vi "Monitoring task.vi"   [LabVIEW 2016]
uses:
  PLC/PLC.lvlib
types:
  T1 = enum16{"启动测量", "标样核查", "零点核查", "跨度核查", "空白测试", "平行样测试", "加标回收", "空白校准", "标样校准", "初始化（清洗）", "停止测试", "仪器重启", "校时", "模式设置", "测量间隔设置"}
  T2 = cluster{"参数启用":cluster{"氨氮":bool, "总磷":bool, "总氮":bool, "多参数":bool, "CODMn":bool, "CODcr":bool, "超标留样":bool}}
  T3 = cluster{"时间标识":timestamp, "设备":string, "日志信息":string, "流程参数":string}
  T4 = cluster{"测量模式":enum16{"水样测量", "标样核查", "零点核查", "跨度核查", "空白测试", "加标回收", "平行样", "校零", "校标"}}
  T5 = cluster{"时间标识":timestamp, "设备":string, "日志信息":string}
  T6 = enum16{"空闲", "水样测试", "标样核查", "零点核查", "跨度核查", "空白测试", "平行样测试", "加标回收", "空白校准", "标样校准", "初始化（清洗）"}
  T7 = cluster{"系统时间":timestamp, "工作状态":u16, "测量模式":enum16{"待机", "连续模式", "周期模式", "定点模式", "受控模式", "手动模式"}, "告警代码":u16, "故障代码":u16, "日志代码":u16, "软件版本":u16, "F0":sgl, "F1":sgl, "F2":sgl, "F3":sgl, "T":sgl, "H":sgl, "id":u16, "flowid":u16, "量程":u16, "总磷控温温度1":sgl, "营养盐控温温度2":sgl, "ADC":sgl}
  T8 = enum16{"空闲", "水样测试", "标样核查", "零点核查", "跨度核查", "空白测试", "平行样测试", "质控样", "空白校准", "标样校准", "加标回收"}
  T9 = enum32{"Bad", "Idle", "Run top level", "Running"}
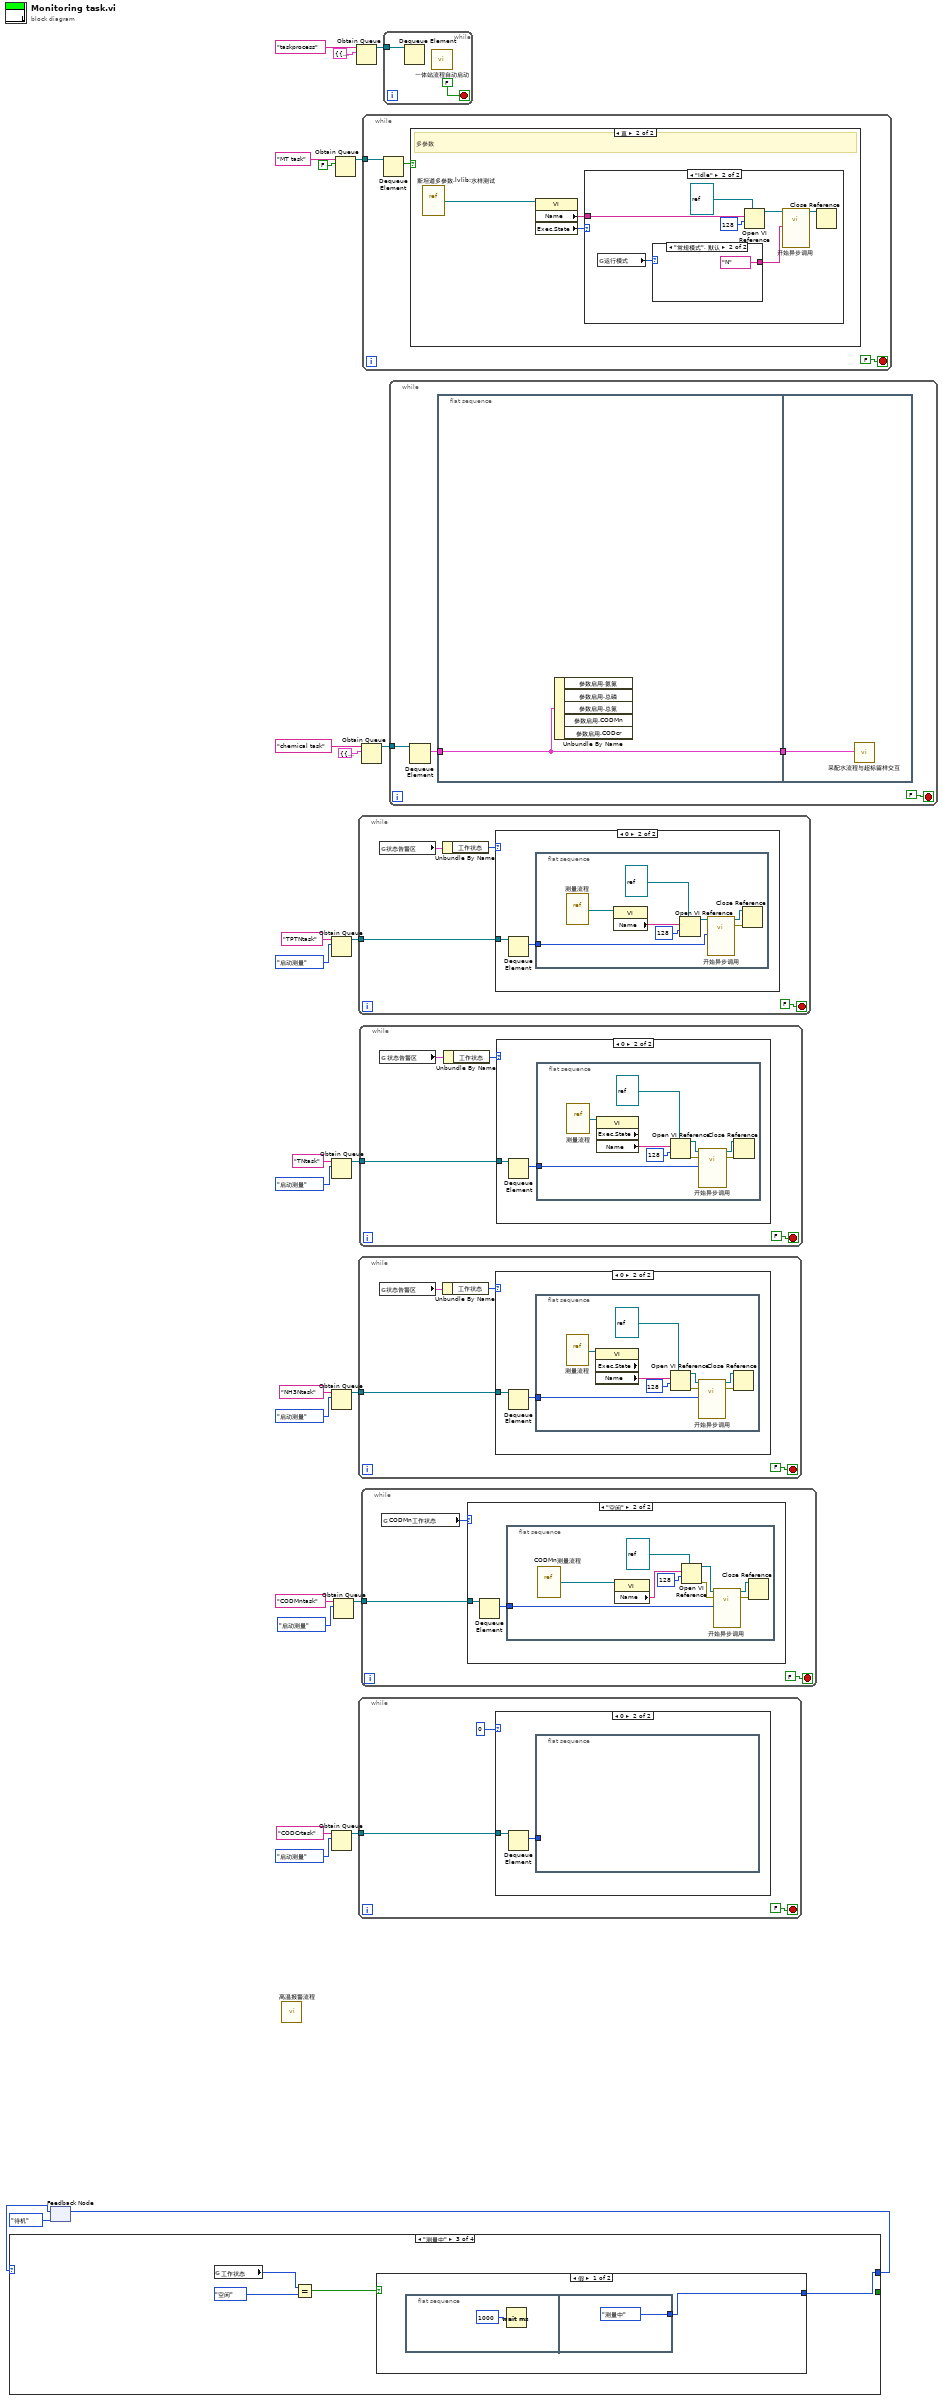
[diagram p0: block diagram]
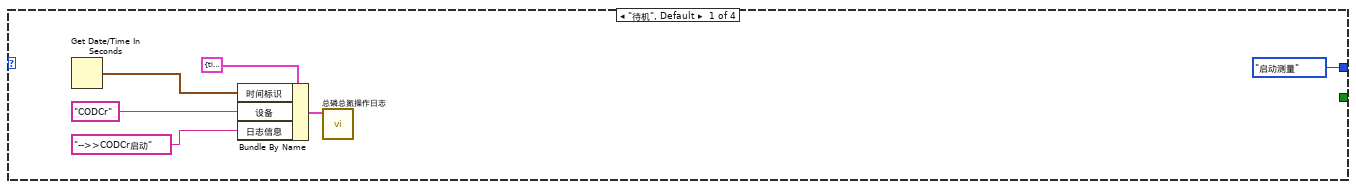
[diagram p2: hidden frame]
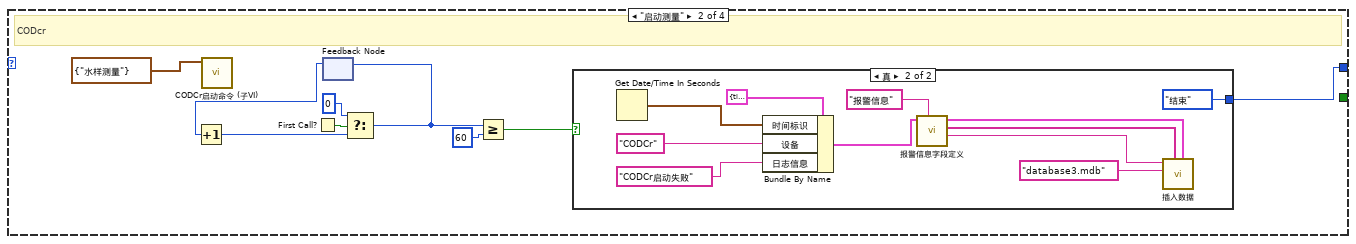
[diagram p3: hidden frame]
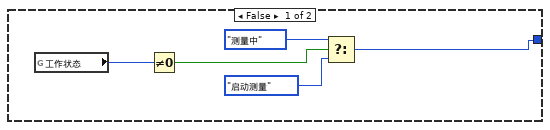
[diagram p4: hidden frame]
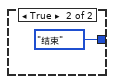
[diagram p5: hidden frame]
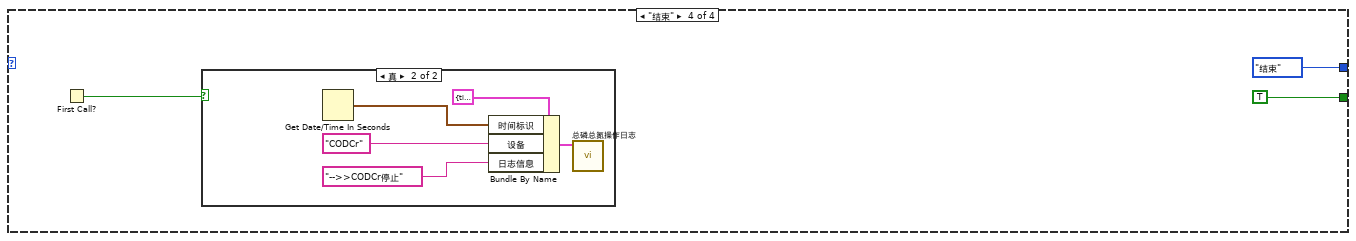
[diagram p6: hidden frame]
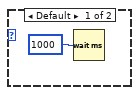
[diagram p8: hidden frame]
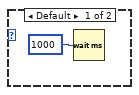
[diagram p9: hidden frame]
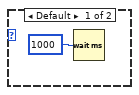
[diagram p10: hidden frame]
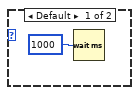
[diagram p11: hidden frame]
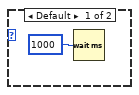
[diagram p12: hidden frame]
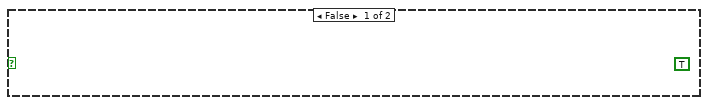
[diagram p13: hidden frame]
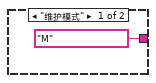
[diagram p15: hidden frame]
diagram:
  n1 = feedback #1(enum16{"待机", "启动测量", "测量中", "结束"}."待机") -> (w2:enum16{"待机", "启动测量", "测量中", "结束"})
  n2 = case shown="\"测量中\"" w2 {
    tunnel: [enum16{"待机", "启动测量", "测量中", "结束"}."启动测量" w42 w62 enum16{"待机", "启动测量", "测量中", "结束"}."结束"] -> w1
    tunnel: [_ _ _ TRUE] -> _
    frame "待机", Default {
      n3 = Get Date/Time In Seconds() -> (seconds since 1Jan1904=w32:timestamp)
      n4 = Bundle By Name(cluster=T3 {"时间标识"=timestamp(0 s since 1904-01-01), "设备"="", "日志信息"="", "流程参数"=""} ("data in"), "时间标识"=w32, "设备"="CODCr", "日志信息"="-->>CODCr启动") -> (w28:T3)
      n5 = call "总磷总氮操作日志.vi"("data in"=w28) -> ()  [unwired: 11 in]
    }
    frame "启动测量" {
      # "CODcr"
      n6 = call "CODCr启动命令 (子VI).vi"("启动测量模式"=T4 {"测量模式"=enum."水样测量"}) -> ()  [unwired: 11 in]
      n7 = First Call?() -> (First Call?: T/F=w37:bool)
      n8 = feedback #2() -> (w38:i32)  [unwired: 1 in]
      n9 = Increment(x=w38) -> (x+1=w39:i32)
      n10 = Select(t=0, s=w37, f=w39) -> (s? t:f=w40:i32)
      n11 = feedback-in #2(w40) -> ()
      n12 = Greater Or Equal?(x=w40, y=60) -> (x >= y?=w35:bool)
      n13 = case shown="真" w35 {
        tunnel: [w43 enum16{"待机", "启动测量", "测量中", "结束"}."结束"] -> w42
        frame False {
          n14 = global read "CODcr全局变量.vi" "工作状态"() -> (w44:T6)
          n15 = Not Equal To 0?(x=w44) -> (x != 0?=w45:bool)
          n16 = Select(t=enum16{"待机", "启动测量", "测量中", "结束"}."测量中", s=w45, f=enum16{"待机", "启动测量", "测量中", "结束"}."启动测量") -> (s? t:f=w43:enum16{"待机", "启动测量", "测量中", "结束"})
        }
        frame True {
          n17 = Get Date/Time In Seconds() -> (seconds since 1Jan1904=w54:timestamp)
          n18 = Bundle By Name(cluster=T5 {"时间标识"=timestamp(0 s since 1904-01-01), "设备"="", "日志信息"=""} ("data in"), "时间标识"=w54, "设备"="CODCr", "日志信息"="CODCr启动失败") -> (w48:T5)
          n19 = call "报警信息字段定义.vi"("table输入"="报警信息", "data in"=w48) -> ("table输出"=w51:string, "columns"=w52:string[], "data out"=w53:T5)  [unwired: 7 in]
          n20 = call "插入数据.vi"("data"=w53, "columns"=w52, "database"="database3.mdb", "table"=w51) -> ()  [unwired: 7 in, 1 out]
        }
      }
    }
    frame "测量中" {
      n21 = global read "CODcr全局变量.vi" "工作状态"() -> (w61:T6)
      n22 = Equal?(x=w61, y=T6."空闲" ("工作状态")) -> (x = y?=w60:bool)
      n23 = case shown="假" w60 {
        tunnel: [w63 enum16{"待机", "启动测量", "测量中", "结束"}."结束"] -> w62
        frame False {
          n24 = flat-sequence {
            tunnel: [enum16{"待机", "启动测量", "测量中", "结束"}."测量中"] -> w63
            frame #0 {
              n25 = Wait (ms)(milliseconds to wait=u32 1000 ("等待时间（毫秒）")) -> ()  [unwired: 1 out]
            }
            frame #1 {
            }
          }
        }
        frame True {
        }
      }
    }
    frame "结束" {
      n26 = First Call?() -> (First Call?: T/F=w67:bool)
      n27 = case shown="真" w67 {
        frame False {
        }
        frame True {
          n28 = Get Date/Time In Seconds() -> (seconds since 1Jan1904=w74:timestamp)
          n29 = Bundle By Name(cluster=T3 {"时间标识"=timestamp(0 s since 1904-01-01), "设备"="", "日志信息"="", "流程参数"=""} ("data in"), "时间标识"=w74, "设备"="CODCr", "日志信息"="-->>CODCr停止") -> (w70:T3)
          n30 = call "总磷总氮操作日志.vi"("data in"=w70) -> ()  [unwired: 11 in]
        }
      }
    }
  }
  n31 = feedback-in #1(w1) -> ()
  n32 = call "高温报警流程.vi"() -> ()  [unwired: 12 in]
  n33 = Obtain Queue(name (unnamed)="TPTNtask" ("名称（未命名）"), element data type=T1."启动测量" ("控制命令")) -> (queue out=w13:refnum<queue>)  [unwired: 3 in, 2 out]
  n34 = Obtain Queue(name (unnamed)="NH3Ntask" ("名称（未命名）"), element data type=T1."启动测量" ("控制命令")) -> (queue out=w12:refnum<queue>)  [unwired: 3 in, 2 out]
  n35 = Obtain Queue(name (unnamed)="CODCrtask" ("名称（未命名）"), element data type=T1."启动测量" ("控制命令")) -> (queue out=w4:refnum<queue>)  [unwired: 3 in, 2 out]
  n36 = Obtain Queue(name (unnamed)="TNtask" ("名称（未命名）"), element data type=T1."启动测量" ("控制命令")) -> (queue out=w16:refnum<queue>)  [unwired: 3 in, 2 out]
  n37 = Obtain Queue(name (unnamed)="CODMntask" ("名称（未命名）"), element data type=T1."启动测量" ("控制命令")) -> (queue out=w7:refnum<queue>)  [unwired: 3 in, 2 out]
  n38 = Obtain Queue(name (unnamed)="MT task" ("名称（未命名）"), element data type=FALSE) -> (queue out=w23:refnum<queue>)  [unwired: 3 in, 2 out]
  n39 = Obtain Queue(name (unnamed)="taskprocess" ("名称（未命名）"), element data type=T2 {"参数启用"={"氨氮"=FALSE, "总磷"=FALSE, "总氮"=FALSE, "多参数"=FALSE, "CODMn"=FALSE, "CODcr"=FALSE, "超标留样"=FALSE}} ("参数")) -> (queue out=w19:refnum<queue>)  [unwired: 3 in, 2 out]
  n40 = while {
    tunnel: w13 -> [w78]
    stop <- FALSE stop-if-true
    n41 = global read "VAR总磷总氮全局变量.vi" "状态告警区"() -> (w76:T7)
    n42 = Unbundle By Name(w76) -> ("工作状态"=w75:u16)
    n43 = case shown="0" w75 {
      tunnel: w78 -> [_ w81]
      frame Default {
        n44 = Wait (ms)(milliseconds to wait=u32 1000 ("等待时间（毫秒）")) -> ()  [unwired: 1 out]
      }
      frame 0 {
        n45 = Dequeue Element(queue=w81) -> (element=w80:T1)  [unwired: 2 in, 3 out]
        n46 = flat-sequence {
          tunnel: w80 -> [w82]
          frame #0 {
            n47 = vi-ref "测量流程.vi"() -> (w87:refnum<vi>)
            n48 = property class="VI"(reference=w87) -> ("Name"=w88:string)  [unwired: 1 in, 2 out]
            n49 = Open VI Reference(type specifier VI Refnum (for type only)=refnum<vi> refnum, vi path=w88, options=128 ("选项")) -> (vi reference=w86:refnum<vi>)  [unwired: 3 in, 1 out]
            n50 = call-by-ref "开始异步调用"(reference=w86, "控制命令"=w82) -> (reference out=w85:refnum<vi>, error out=w84:errorcluster)  [unwired: 12 in]
            n51 = Close Reference(reference=w85, error in (no error)=w84) -> ()  [unwired: 1 out]
          }
        }
      }
    }
  }
  n52 = while {
    tunnel: w12 -> [w93]
    stop <- FALSE stop-if-true
    n53 = global read "VAR总磷总氮全局变量.vi" "状态告警区"() -> (w91:T7)
    n54 = Unbundle By Name(w91) -> ("工作状态"=w90:u16)
    n55 = case shown="0" w90 {
      tunnel: w93 -> [_ w96]
      frame Default {
        n56 = Wait (ms)(milliseconds to wait=u32 1000 ("等待时间（毫秒）")) -> ()  [unwired: 1 out]
      }
      frame 0 {
        n57 = Dequeue Element(queue=w96) -> (element=w95:T1)  [unwired: 2 in, 3 out]
        n58 = flat-sequence {
          tunnel: w95 -> [w97]
          frame #0 {
            n59 = vi-ref "测量流程.vi"() -> (w105:refnum<vi>)
            n60 = property class="VI" props=["Exec.State", "Name"](reference=w105) -> ("Name"=w104:string)  [unwired: 1 in, 3 out]
            n61 = Open VI Reference(type specifier VI Refnum (for type only)=refnum<vi> refnum, vi path=w104, options=128 ("选项")) -> (vi reference=w99:refnum<vi>, error out=w101:errorcluster)  [unwired: 3 in]
            n62 = call-by-ref "开始异步调用"(reference=w99, error in=w101, "控制命令"=w97) -> (reference out=w102:refnum<vi>, error out=w103:errorcluster)  [unwired: 11 in]
            n63 = Close Reference(reference=w102, error in (no error)=w103) -> ()  [unwired: 1 out]
          }
        }
      }
    }
  }
  n64 = while {
    tunnel: w4 -> [w108]
    stop <- FALSE stop-if-true
    n65 = case shown="0" u16 0 ("工作状态") {
      tunnel: w108 -> [_ w111]
      frame Default {
        n66 = Wait (ms)(milliseconds to wait=u32 1000 ("等待时间（毫秒）")) -> ()  [unwired: 1 out]
      }
      frame 0 {
        n67 = Dequeue Element(queue=w111) -> (element=w110:T1)  [unwired: 2 in, 3 out]
        n68 = flat-sequence {
          tunnel: w110 -> [_]
          frame #0 {
          }
        }
      }
    }
  }
  n69 = while {
    tunnel: w16 -> [w115]
    stop <- FALSE stop-if-true
    n70 = global read "VAR总磷总氮全局变量.vi" "状态告警区"() -> (w113:T7)
    n71 = Unbundle By Name(w113) -> ("工作状态"=w112:u16)
    n72 = case shown="0" w112 {
      tunnel: w115 -> [_ w118]
      frame Default {
        n73 = Wait (ms)(milliseconds to wait=u32 1000 ("等待时间（毫秒）")) -> ()  [unwired: 1 out]
      }
      frame 0 {
        n74 = Dequeue Element(queue=w118) -> (element=w117:T1)  [unwired: 2 in, 3 out]
        n75 = flat-sequence {
          tunnel: w117 -> [w127]
          frame #0 {
            n76 = vi-ref "测量流程.vi"() -> (w126:refnum<vi>)
            n77 = property class="VI" props=["Exec.State", "Name"](reference=w126) -> ("Name"=w125:string)  [unwired: 1 in, 3 out]
            n78 = Open VI Reference(type specifier VI Refnum (for type only)=refnum<vi> refnum, vi path=w125, options=128 ("选项")) -> (vi reference=w120:refnum<vi>, error out=w122:errorcluster)  [unwired: 3 in]
            n79 = call-by-ref "开始异步调用"(reference=w120, error in=w122, "控制命令"=w127) -> (reference out=w123:refnum<vi>, error out=w124:errorcluster)  [unwired: 11 in]
            n80 = Close Reference(reference=w123, error in (no error)=w124) -> ()  [unwired: 1 out]
          }
        }
      }
    }
  }
  n81 = while {
    tunnel: w7 -> [w130]
    stop <- FALSE stop-if-true
    n82 = global read "COD测量模式全局.vi" "CODMn工作状态"() -> (w128:T8)
    n83 = case shown="\"空闲\"" w128 {
      tunnel: w130 -> [_ w133]
      frame Default {
        n84 = Wait (ms)(milliseconds to wait=u32 1000 ("等待时间（毫秒）")) -> ()  [unwired: 1 out]
      }
      frame "空闲" {
        n85 = Dequeue Element(queue=w133) -> (element=w132:T1)  [unwired: 2 in, 3 out]
        n86 = flat-sequence {
          tunnel: w132 -> [w134]
          frame #0 {
            n87 = vi-ref "CODMn测量流程.vi"() -> (w141:refnum<vi>)
            n88 = property class="VI"(reference=w141) -> ("Name"=w142:string)  [unwired: 1 in, 2 out]
            n89 = Open VI Reference(type specifier VI Refnum (for type only)=refnum<vi> refnum, vi path=w142, options=128 ("选项")) -> (vi reference=w136:refnum<vi>, error out=w138:errorcluster)  [unwired: 3 in]
            n90 = call-by-ref "开始异步调用"(reference=w136, error in=w138, "控制命令"=w134) -> (reference out=w139:refnum<vi>, error out=w140:errorcluster)  [unwired: 11 in]
            n91 = Close Reference(reference=w139, error in (no error)=w140) -> ()  [unwired: 1 out]
          }
        }
      }
    }
  }
  n92 = Obtain Queue(name (unnamed)="chemical task" ("名称（未命名）"), element data type=T2 {"参数启用"={"氨氮"=FALSE, "总磷"=FALSE, "总氮"=FALSE, "多参数"=FALSE, "CODMn"=FALSE, "CODcr"=FALSE, "超标留样"=FALSE}} ("参数")) -> (queue out=w25:refnum<queue>)  [unwired: 3 in, 2 out]
  n93 = while {
    tunnel: w23 -> [w145]
    stop <- FALSE stop-if-true
    n94 = Dequeue Element(queue=w145) -> (element=w144:bool)  [unwired: 2 in, 3 out]
    n95 = case shown="真" w144 {
      frame False {
        (unwired) TRUE ("t")
      }
      frame True {
        # "多参数"
        n96 = vi-ref "斯坦道多参数.lvlib:水样测试.vi"() -> (w147:refnum<vi>)
        n97 = property class="VI"(reference=w147) -> ("Name"=w146:string, "Exec.State"=w148:T9)  [unwired: 1 in, 2 out]
        n98 = case shown="\"Idle\"" w148 {
          tunnel: w146 -> [_ w155]
          frame "Bad", Default {
          }
          frame "Idle" {
            n99 = global read "系统设置全局变量.vi" "运行模式"() -> (w150:enum16{"维护模式", "常规模式", "应急模式", "质控模式"})
            n100 = case shown="\"常规模式\", 默认" w150 {
              tunnel: ["M" ("数据标记表") "N" ("数据标记表")] -> w151
              frame "维护模式" {
              }
              frame "常规模式", Default {
              }
            }
            n101 = Open VI Reference(type specifier VI Refnum (for type only)=refnum<vi> refnum, vi path=w155, options=128 ("选项")) -> (vi reference=w153:refnum<vi>)  [unwired: 3 in, 1 out]
            n102 = call-by-ref "开始异步调用"(reference=w153, "数据标记表"=w151) -> (reference out=w152:refnum<vi>)  [unwired: 12 in, 1 out]
            n103 = Close Reference(reference=w152) -> ()  [unwired: 1 in, 1 out]
          }
        }
      }
    }
  }
  n104 = while {
    tunnel: w19 -> [w159]
    stop <- FALSE stop-if-true
    n105 = Dequeue Element(queue=w159) -> ()  [unwired: 2 in, 4 out]
    n106 = call "一体站流程自动启动.vi"() -> ()  [unwired: 12 in]
  }
  n107 = while {
    tunnel: w25 -> [w162]
    stop <- FALSE stop-if-true
    n108 = Dequeue Element(queue=w162) -> (element=w161:T2)  [unwired: 2 in, 3 out]
    n109 = flat-sequence {
      tunnel: [w164] -> w163
      tunnel: w161 -> [w164]
      tunnel: w163 -> [w165]
      frame #0 {
        n110 = Unbundle By Name(w164) -> ()  [unwired: 5 out]
      }
      frame #1 {
        n111 = call "采配水流程与超标留样交互.vi"("参数"=w165) -> ()  [unwired: 11 in]
      }
    }
  }
